vi "20查看高雄市.vi"() -> ()   [LabVIEW 2014]
panel:
  in  "OK Button":bool
  in  "底色":u32(colorbox)=16768479
  # "高雄市"
  # "土地價格：1800"
  # "高\n雄\n發\n大\n財\n!!"
  # "高\n雄\n發\n大\n財\n!!"
  # "蓋房子價格：850"
  # "蓋旅館價格：1500"
  # "過路費"
  # "空地：300"
  # "一棟房子：+450"
  # "一棟旅館：+1000"
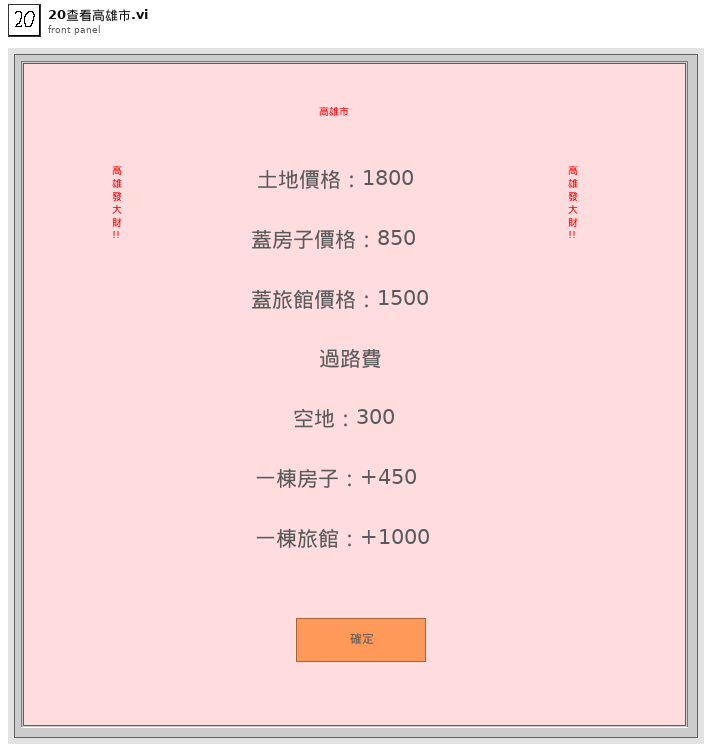
[diagram p1: front panel]
types:
  T1 = enum8{"Enabled", "Disabled", "Disabled and Grayed Out"}
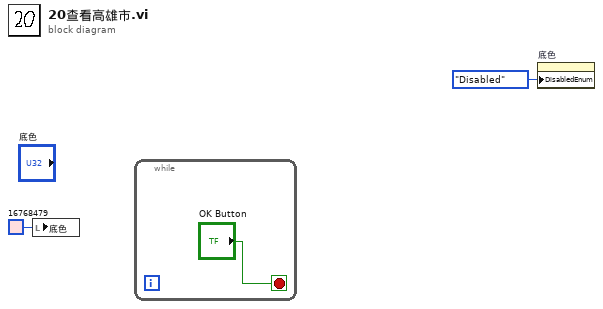
[diagram p0: block diagram]
diagram:
  n1 = local write "底色"(u32 16768479 ("底色")) -> ()
  n2 = while {
    stop <- "OK Button" stop-if-true
  }
  n3 = property on="底色" class="ColBox"("DisabledEnum"=T1."Disabled" ("Disabled")) -> ()  [unwired: 2 in, 2 out]
